vi "Run Test (Object).vi"(5 "Test Report":refnum<class "Test Report.lvclass">, 6 "Verbose":bool, 7 "Report Path":path, 8 "error in":errorcluster, 10 "Object":refnum<class>, 11 "Interactive (T)":bool=TRUE) -> (0 "error out":errorcluster)   [LabVIEW 2013, in "Caraya.lvlib"]
uses:
  classes/Test Report/Test Report.lvclass
  <userlib>/_OpenG.lib/file/file.llb/Strip Path Extension - Path__ogtk.vi
  classes/Test Runner.Folder/Test Runner.Folder.lvclass
  Caraya.lvlib
  classes/Test Runner/Test Runner.lvclass
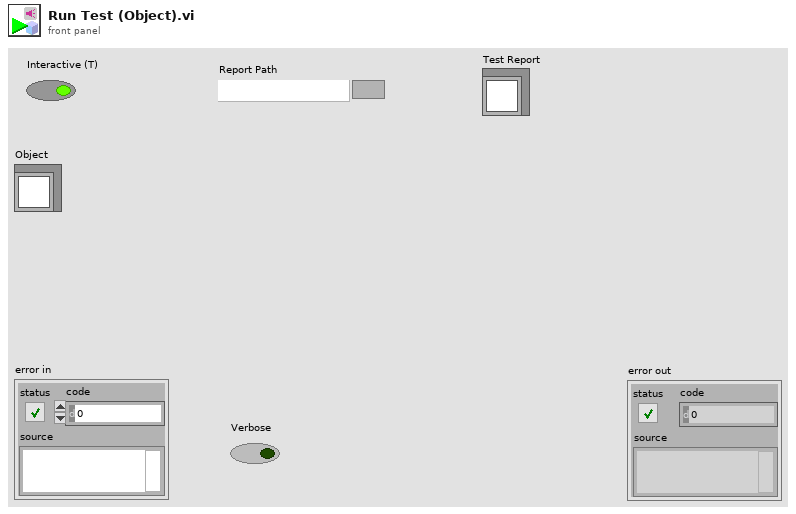
[diagram p1: front panel]
types:
  T1 = enum32{"invalid scope", "public", "private", "protected", "community"}
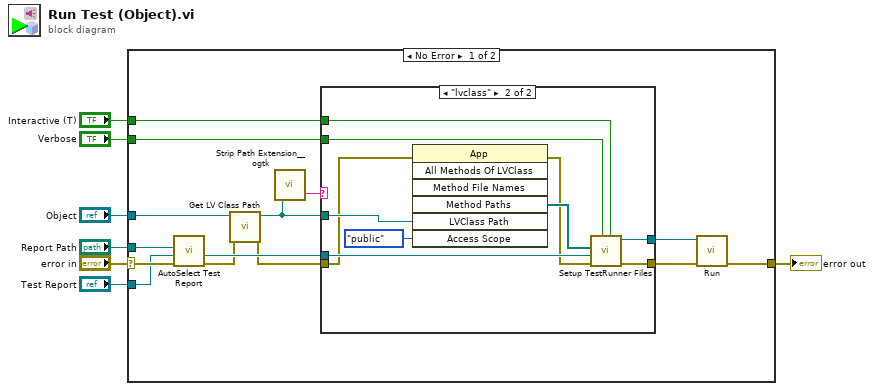
[diagram p0: block diagram]
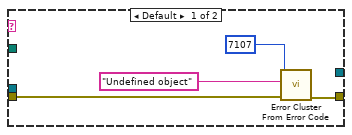
[diagram p2: hidden frame]
diagram:
  n1 = case shown="No Error" "error in" {
    selector: "error in" -> [w18 w36]
    tunnel: [w21 w36] -> w7
    tunnel: "Verbose" -> [w20 _]
    tunnel: "Interactive (T)" -> [w19 _]
    tunnel: "Test Report" -> [w16 _]
    tunnel: "Object" -> [w14 _]
    tunnel: "Report Path" -> [w17 _]
    frame No Error {
      n2 = call "AutoSelect Test Report.vi"("error in (no error)"=w18, "Test Report in"=w16, "Report Path"=w17) -> ("error out"=w9:errorcluster, "Test Report out"=w15:refnum<class "Test Report.lvclass">)  [unwired: 7 in]
      n3 = call <vilib>:"Get LV Class Path.vi"("error in (no error)"=w9, "object"=w14) -> ("error out"=w8:errorcluster, "class path"=w13:path)  [unwired: 8 in]
      n4 = call-poly <userlib>:"Strip Path Extension__ogtk.vi"("path"=w13) -> ("extension"=w10:string)  [unwired: 1 out]
      n5 = case shown="\"lvclass\"" w10 {
        tunnel: w8 -> [w23 w27]
        tunnel: [w22 w35] -> w12
        tunnel: [_ w34] -> w11
        tunnel: w19 -> [_ w33]
        tunnel: w20 -> [_ w32]
        tunnel: w15 -> [_ w31]
        tunnel: w13 -> [_ w29]
        frame Default {
          n6 = call <vilib>:"Error Cluster From Error Code.vi"("error in (no error)"=w23, "error message (\"\")"="Undefined object" ("error message (\"\")"), "error code (0)"=7107 ("code")) -> ("error out"=w22:errorcluster)  [unwired: 6 in]
        }
        frame "lvclass" {
          n7 = invoke class="App" method="All Methods Of LVClass"(error in=w27, "LVClass Path"=w29, "Access Scope"=T1."public") -> (error out=w26:errorcluster, "Method Paths"=w28:path[])  [unwired: 4 in, 5 out]
          n8 = call "Setup TestRunner Files.vi"("Interactive (T)"=w33, "Verbose (F)"=w32, "error in (no error)"=w26, "Test Report"=w31, "Paths"=w28) -> ("error out"=w35:errorcluster, "Test Runner.Folder out"=w34:refnum<class "Test Runner.Folder.lvclass">)  [unwired: 5 in]
        }
      }
      n9 = call "Run.vi"("error in (no error)"=w12, "Test Runner in"=w11) -> ("error out"=w21:errorcluster)  [unwired: 8 in, 1 out]
    }
    frame Error {
    }
  }
  "error out" <- w7
